vi "Seq Dialog ParemeterSet2.0.vi"(8 "Segment Data":T1) -> (0 "Step Hisitory":string[](array[string]), 2 "Segment Data 2":T1)   [LabVIEW 2018]
uses:
  type defs/Sequence Info.ctl
  type defs/17x Audit Motion Data Seq Control.ctl
  type defs/17x AP Data Type.ctl
panel:
  out "String":string="Pre Run Station - Glass - Vent Open"
  out "error out":errorcluster
  out "value":T2={"Power Supply Voltage"=0.0, "Min Avg Current"=0.0, "Max Avg Current"=0.0, "Min Run Time"=0.0, "Max Run Time"=0.0, "Min Speed"=0.0, "Max Speed"=0.0, "AP Data % of Threshold"=10.0, "Travel Distance"=0.0, "AP Data Type"=enum."91/61", "Check Current"=FALSE, "Check Run Time"=FALSE, "Check Speed"=FALSE, "Express Motion?"=FALSE, "Check Sound Test"=FALSE, "Check Position?"=FALSE, "Collect AP Data"=FALSE, "Inital Position"=0, "End Position"=0, "Goto Posiition"=0, "Max max Current"=0.0, "Min max Current"=0.0, "Check max Current"=FALSE, "Check Sound"=FALSE, "Min Sound (dB)"=0.0, "Max Sound (dB)"=0.0, "SW Mode"=enum."Hard Switch", "LIN Msg"={"ID"=0, "Msg"=[], "LDF"="EX1H"}} {"LIN Msg"."Msg" format="%02x"; "LIN Msg"."ID" format="%02x"}
  in  "Description":string
  in  "Save":bool
  in  "Cancel":bool
  in  "Goto Position":u16=133 max=6750
  in  "FullClose Position":u16=133 min=80 max=6750
  in  "FullOpen Position":u16=133 min=80 max=6750
  in  "Check max Current":bool
  in  "Max max Current (amps)":dbl=10.0
  in  "Min max Current (amps)":dbl=10.0
  in  "Max Speed (mm/sec)":dbl=10.0
  in  "Min Speed (mm/sec)":dbl=10.0
  in  "Check Speed":bool
  in  "Travel Distance (mm)":dbl=133.0
  in  "Check Current":bool
  in  "Check Run Time":bool
  in  "Max Run Time (secs)":dbl=10.0
  in  "Min Run Time (secs)":dbl=10.0
  in  "Max Avg Current (amps)":dbl=10.0
  in  "Min Avg Current (amps)":dbl=10.0
  in  "Power Supply Voltage (V)":dbl=13.0
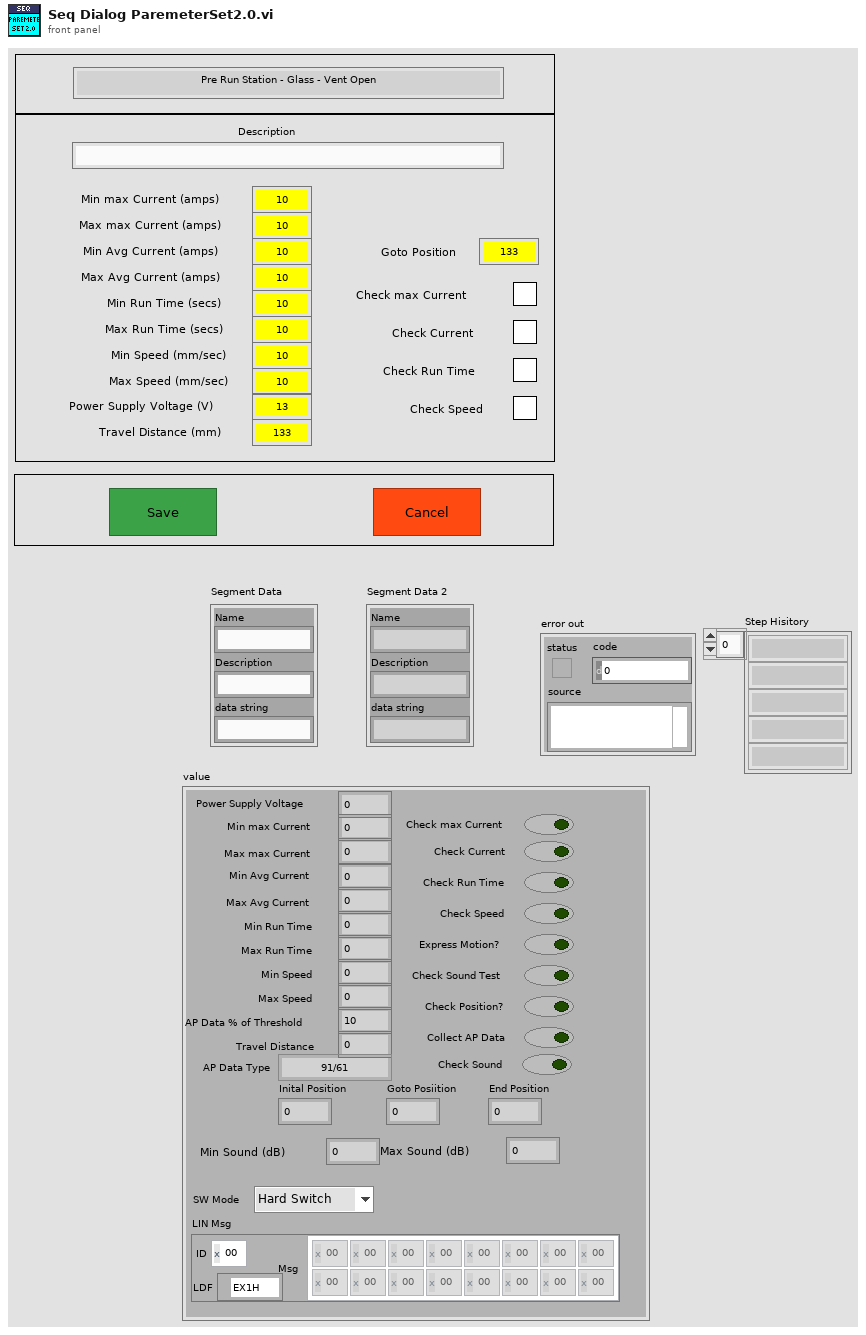
[diagram p1: front panel]
types:
  T1 = typedef "Sequence Info.ctl" = cluster{"Name":string, "Description":string, "data string":string}
  T2 = typedef "17x Audit Motion Data Seq Control.ctl" = cluster{"Power Supply Voltage":dbl, "Min Avg Current":dbl, "Max Avg Current":dbl, "Min Run Time":dbl, "Max Run Time":dbl, "Min Speed":dbl, "Max Speed":dbl, "AP Data % of Threshold":dbl, "Travel Distance":dbl, "AP Data Type":T3, "Check Current":bool, "Check Run Time":bool, "Check Speed":bool, "Express Motion?":bool, "Check Sound Test":bool, "Check Position?":bool, "Collect AP Data":bool, "Inital Position":u16, "End Position":u16, "Goto Posiition":u16, "Max max Current":dbl, "Min max Current":dbl, "Check max Current":bool, "Check Sound":bool, "Min Sound (dB)":dbl, "Max Sound (dB)":dbl, "SW Mode":enum16{"Hard Switch", "Uncond Frame"}, "LIN Msg":cluster{"ID":u8, "Msg":u8[][], "LDF":refnum<k21>}}
  T3 = typedef "17x AP Data Type.ctl" = enum16{"91/61", "92/62", "93/63", "67", "68", "6F", "71", "91 Msg", "92 Msg", "93 Msg", "94 Msg", "HiRain 91", "HiRain 92 Speed", "HiRain 92 HS", "HiRain 92", "HiRain 93", "SnT"}
  T4 = cluster{"Hall Positions":i32[], "Hall path":path, "Motion Data Cluster":T2, "Segment Data":T1, "Old Data":string, "New Data":string}
  T5 = typedef "config paths for seq def.ctl" = cluster{"Part Type":string, "base path":path}
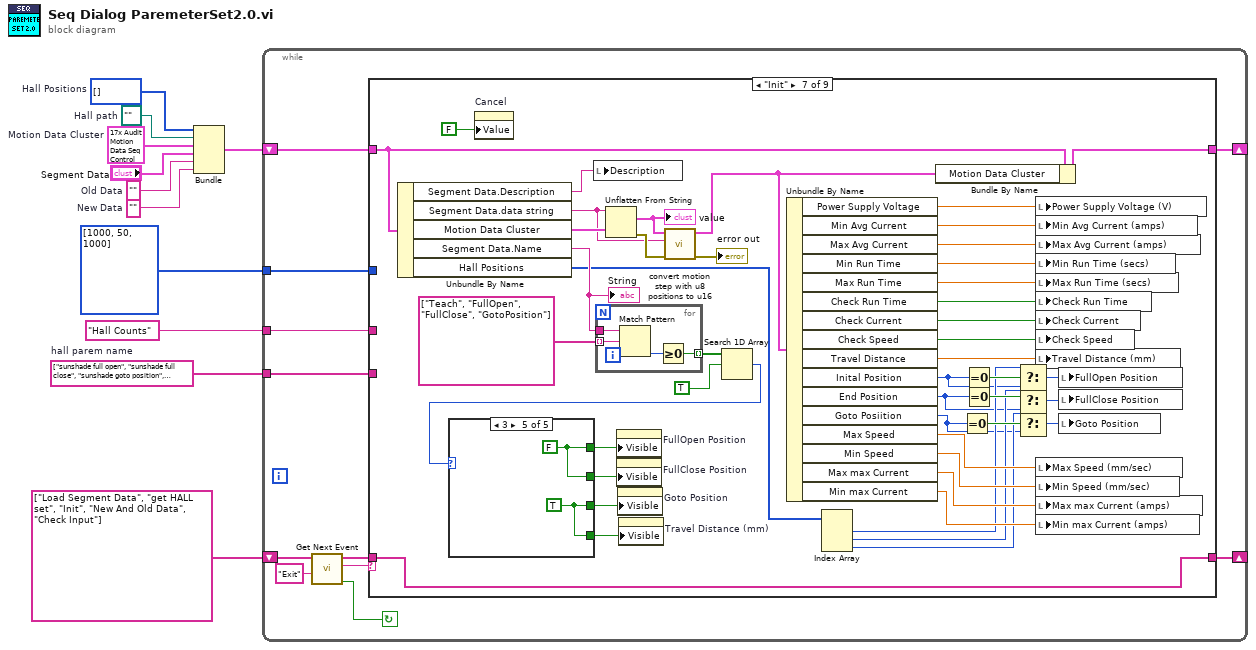
[diagram p0: block diagram]
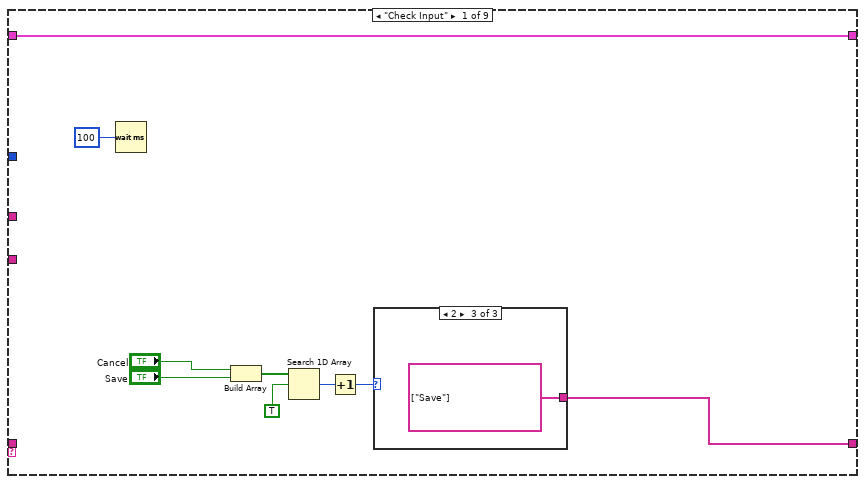
[diagram p2: hidden frame]
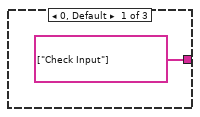
[diagram p3: hidden frame]
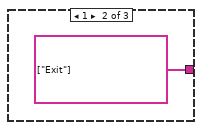
[diagram p4: hidden frame]
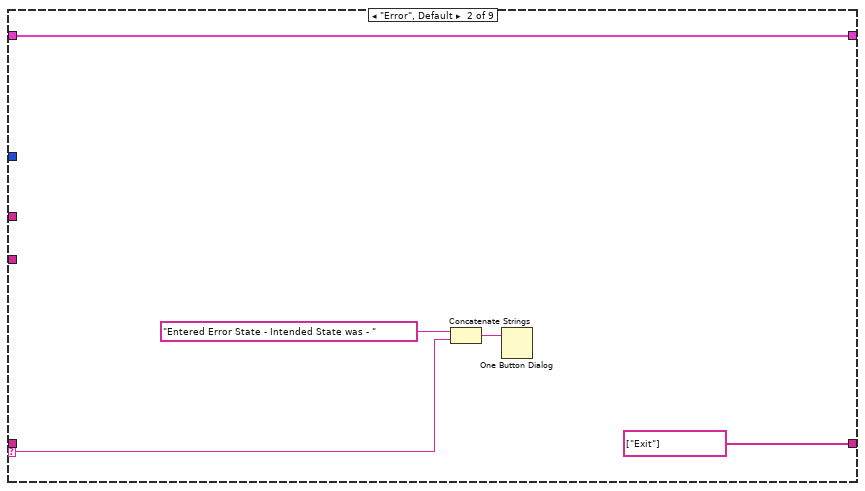
[diagram p5: hidden frame]
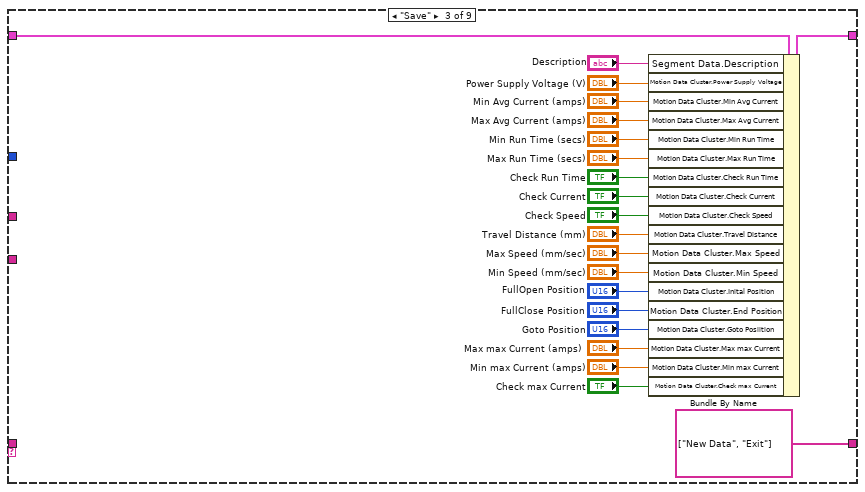
[diagram p6: hidden frame]
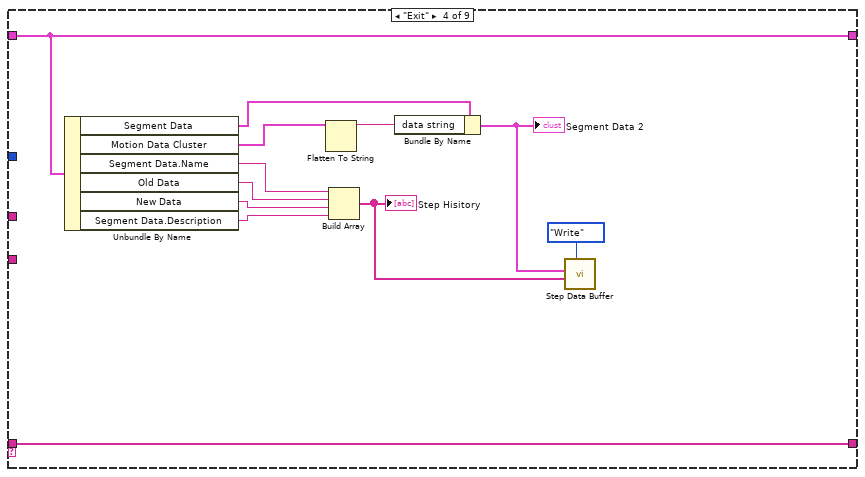
[diagram p7: hidden frame]
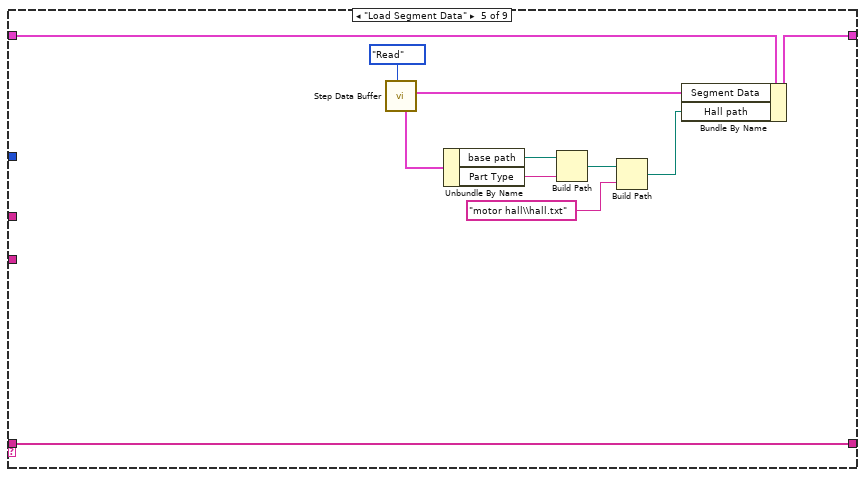
[diagram p8: hidden frame]
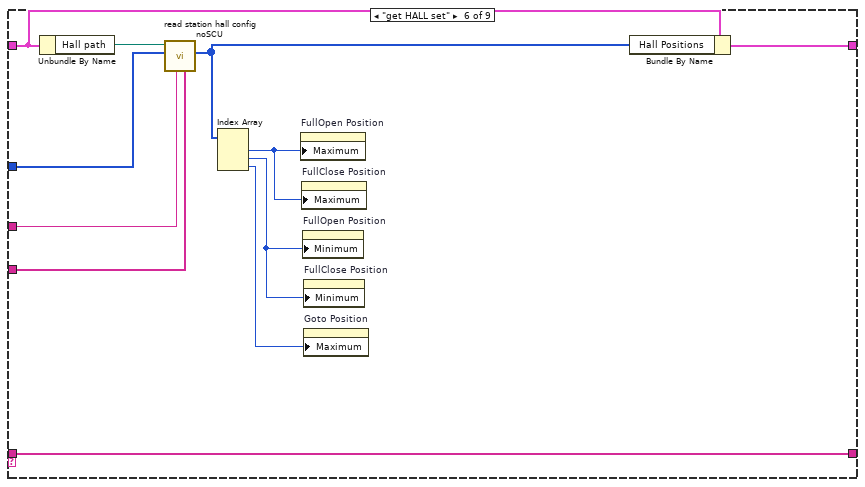
[diagram p9: hidden frame]
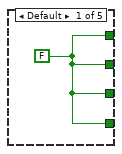
[diagram p10: hidden frame]
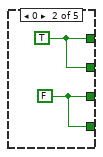
[diagram p11: hidden frame]
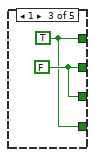
[diagram p12: hidden frame]
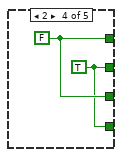
[diagram p13: hidden frame]
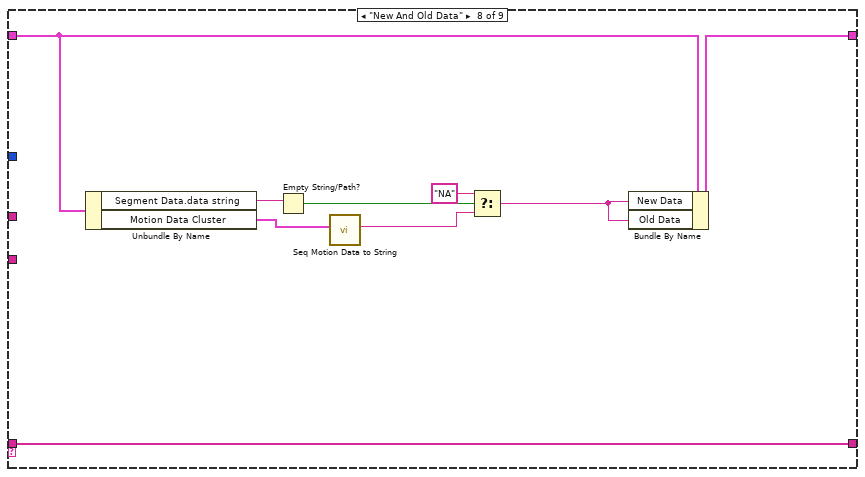
[diagram p14: hidden frame]
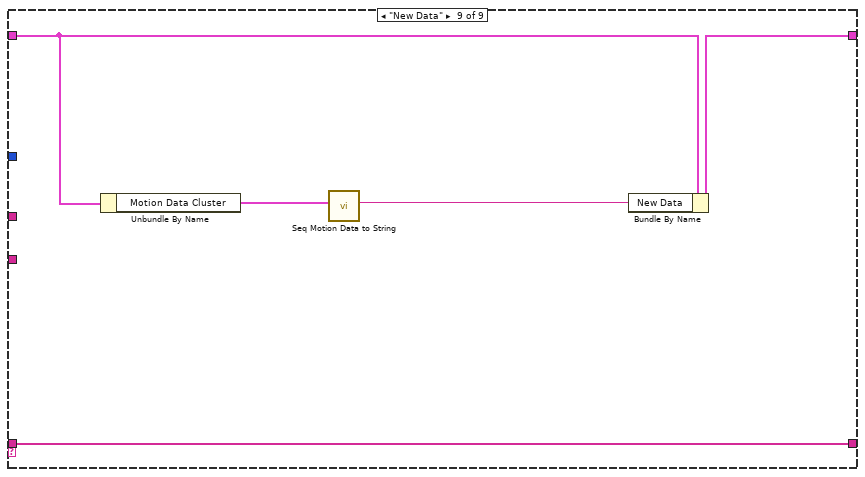
[diagram p15: hidden frame]
diagram:
  w5 = path ""  # Hall path
  w1 = string[] ["sunshade full open", "sunshade full close", "sunshade goto position", "sunshade open drift offset", "sunshade close drift offset", "sunshade goto position drift offset"]  # hall parem name
  w4 = i32[] []  # Hall Positions
  w10 = T2 {"Power Supply Voltage"=0.0, "Min Avg Current"=0.0, "Max Avg Current"=0.0, "Min Run Time"=0.0, "Max Run Time"=0.0, "Min Speed"=0.0, "Max Speed"=0.0, "AP Data % of Threshold"=0.0, "Travel Distance"=0.0, "AP Data Type"=enum."91/61", "Check Current"=FALSE, "Check Run Time"=FALSE, "Check Speed"=FALSE, "Express Motion?"=FALSE, "Check Sound Test"=FALSE, "Check Position?"=FALSE, "Collect AP Data"=FALSE, "Inital Position"=0, "End Position"=0, "Goto Posiition"=0, "Max max Current"=0.0, "Min max Current"=0.0, "Check max Current"=FALSE, "Check Sound"=FALSE, "Min Sound (dB)"=0.0, "Max Sound (dB)"=0.0, "SW Mode"=enum."Hard Switch", "LIN Msg"={"ID"=0, "Msg"=[], "LDF"="EX1H"}}  # Motion Data Cluster
  w7 = ""  # New Data
  w8 = ""  # Old Data
  n1 = Bundle("Hall Positions"=w4, "Hall path"=w5, "Motion Data Cluster"=w10, "Segment Data"="Segment Data", "Old Data"=w8, "New Data"=w7) -> (w11:T4)  [unwired: 1 in]
  n2 = while {
    shift-right: [w20] -> _
    shift-left: string[] ["Load Segment Data", "get HALL set", "Init", "New And Old Data", "Check Input"] ("Event queue out") -> [w19]
    shift-right: [w15] -> _
    shift-left: w11 -> [w16]
    tunnel: i32[] [1000, 50, 1000] ("Hall Positions") -> [w14]
    tunnel: "Hall Counts" ("section") -> [w13]
    tunnel: w1 -> [w12]
    stop <- w18 continue-if-true
    n3 = call "Get Next Event.vi"("Exit Event"="Exit", "event queue in"=w19) -> ("Condition (Exit:F)"=w18:bool, "next event"=w22:string, "event queue out"=w21:string[])  [unwired: 3 in]
    n4 = case shown="\"Init\"" w22 {
      selector: w22 -> [_ w36 _ _ _ _ _ _ _]
      tunnel: w21 -> [_ _ _ w72 w82 w84 w96 w162 w167]
      tunnel: [w25 string[] ["Exit"] ("event queue out") string[] ["New Data", "Exit"] ("Event queue out") w72 w82 w84 w96 w162 w167] -> w20
      tunnel: w16 -> [w31 w35 w60 w68 w81 w92 w138 w157 w166]
      tunnel: [w31 w35 w59 w68 w80 w90 w137 w156 w165] -> w15
      tunnel: w14 -> [_ _ _ _ _ w93 _ _ _]
      tunnel: w13 -> [_ _ _ _ _ w86 _ _ _]
      tunnel: w12 -> [_ _ _ _ _ w85 _ _ _]
      frame "Check Input" {
        n5 = Wait (ms)(milliseconds to wait=u32 100) -> ()  [unwired: 1 out]
        n6 = Build Array("Cancel", "Save") -> (w27:bool[])
        n7 = Search 1D Array(1D array=w27, element=TRUE) -> (index of element=w28:i32)  [unwired: 1 in]
        n8 = Increment(x=w28) -> (x+1=w29:i32)
        n9 = case shown="2" w29 {
          tunnel: [string[] ["Check Input"] ("Events to Insert") string[] ["Exit"] ("Events to Insert") string[] ["Save"] ("Events to Insert")] -> w25
          frame 0, Default {
          }
          frame 1 {
          }
          frame 2 {
          }
        }
      }
      frame "Error", Default {
        n10 = Concatenate Strings("Entered Error State - Intended State was - " ("string"), w36) -> (w38:string)
        n11 = One Button Dialog(message=w38) -> ()  [unwired: 1 in, 1 out]
      }
      frame "Save" {
        n12 = Bundle By Name(cluster=w60, "Segment Data.Description"="Description", "Motion Data Cluster.Power Supply Voltage"="Power Supply Voltage (V)", "Motion Data Cluster.Min Avg Current"="Min Avg Current (amps)", "Motion Data Cluster.Max Avg Current"="Max Avg Current (amps)", "Motion Data Cluster.Min Run Time"="Min Run Time (secs)", "Motion Data Cluster.Max Run Time"="Max Run Time (secs)", "Motion Data Cluster.Check Run Time"="Check Run Time", "Motion Data Cluster.Check Current"="Check Current", "Motion Data Cluster.Check Speed"="Check Speed", "Motion Data Cluster.Travel Distance"="Travel Distance (mm)", "Motion Data Cluster.Max Speed"="Max Speed (mm/sec)", "Motion Data Cluster.Min Speed"="Min Speed (mm/sec)", "Motion Data Cluster.Inital Position"="FullOpen Position", "Motion Data Cluster.End Position"="FullClose Position", "Motion Data Cluster.Goto Posiition"="Goto Position", "Motion Data Cluster.Max max Current"="Max max Current (amps)", "Motion Data Cluster.Min max Current"="Min max Current (amps)", "Motion Data Cluster.Check max Current"="Check max Current") -> (w59:T4)
      }
      frame "Exit" {
        n13 = Unbundle By Name(w68) -> ("Segment Data"=w66:T1, "Motion Data Cluster"=w67:T2, "Segment Data.Name"=w70:string, "Old Data"=w69:string, "New Data"=w71:string, "Segment Data.Description"=w61:string)
        n14 = Flatten To String(anything=w67) -> (data string=w65:string)  [unwired: 3 in, 2 out]
        n15 = Build Array(w70, w69, w71, w61) -> (w62:string[])
        "Step Hisitory" <- w62
        n16 = Bundle By Name(cluster=w66, "data string"=w65) -> (w63:T1)
        "Segment Data 2" <- w63
        n17 = call "Step Data Buffer.vi"("Mode"=enum16{"Init", "Read", "Write"}."Write", "Step Hisitory In"=w62, "Segment Data In"=w63) -> ()  [unwired: 4 in, 5 out]
      }
      frame "Load Segment Data" {
        n18 = call "Step Data Buffer.vi"("Mode"=enum16{"Init", "Read", "Write"}."Read") -> ("Segment Data Out"=w79:T1, "config paths"=w74:T5)  [unwired: 6 in, 3 out]
        n19 = Unbundle By Name(w74) -> ("base path"=w78:path, "Part Type"=w77:string)
        n20 = Build Path(base path=w78, name or relative path=w77) -> (appended path=w76:path)
        n21 = Build Path(base path=w76, name or relative path="motor hall\\hall.txt" ("名称或相对路径")) -> (appended path=w73:path)
        n22 = Bundle By Name(cluster=w81, "Segment Data"=w79, "Hall path"=w73) -> (w80:T4)
      }
      frame "get HALL set" {
        n23 = Unbundle By Name(w92) -> ("Hall path"=w94:path)
        n24 = call "read station hall config noSCU.vi"("name"=w85, "section"=w86, "default value"=w93, "configuration file path in"=w94) -> ("Hall Positions"=w91:i32[])  [unwired: 4 in, 3 out]
        n25 = Index Array(array=w91) -> (element #1=w89:i32, element #2=w88:i32, element #3=w87:i32)  [unwired: 3 in]
        n26 = property on="FullOpen Position" class="DigNum (严格)"("Maximum"=w89) -> ()  [unwired: 2 in, 2 out]
        n27 = property on="FullClose Position" class="DigNum (严格)"("Maximum"=w89) -> ()  [unwired: 2 in, 2 out]
        n28 = property on="FullOpen Position" class="DigNum (严格)"("Minimum"=w88) -> ()  [unwired: 2 in, 2 out]
        n29 = property on="FullClose Position" class="DigNum (严格)"("Minimum"=w88) -> ()  [unwired: 2 in, 2 out]
        n30 = property on="Goto Position" class="DigNum (严格)"("Maximum"=w87) -> ()  [unwired: 2 in, 2 out]
        n31 = Bundle By Name(cluster=w92, "Hall Positions"=w91) -> (w90:T4)
      }
      frame "Init" {
        n32 = Unbundle By Name(w138) -> ("Segment Data.Description"=w139:string, "Segment Data.data string"=w122:string, "Motion Data Cluster"=w140:T2, "Segment Data.Name"=w117:string, "Hall Positions"=w109:i32[])
        "String" <- w117
        n33 = property on="Cancel" class="Bool (严格)"("Value"=FALSE ("Cancel")) -> ()  [unwired: 2 in, 2 out]
        n34 = local write "Description"(w139) -> ()
        n35 = for {
          tunnel: w117 -> [w153]
          tunnel: string[] ["Teach", "FullOpen", "FullClose", "GotoPosition"] -> [w152] mode=indexing
          tunnel: [w150] -> w115 mode=indexing
          n36 = Match Pattern(string=w153, regular expression=w152) -> (offset past match=w151:i32)  [unwired: 1 in, 3 out]
          n37 = Greater Or Equal To 0?(x=w151) -> (x >= 0?=w150:bool)
        }
        n38 = Unflatten From String(type=w140, binary string=w122) -> (value=w121:T2, error out=w124:errorcluster)  [unwired: 3 in, 1 out]
        "value" <- w121
        n39 = call "convert motion step with u8 positions to u16.vi"("error in"=w124, "data string"=w122, "Motion Data Cluster in"=w121) -> ("error out"=→"error out":errorcluster, "Motion Data Cluster out"=w120:T2)  [unwired: 7 in]
        n40 = Search 1D Array(1D array=w115, element=TRUE ("元素")) -> (index of element=w113:i32)  [unwired: 1 in]
        n41 = case shown="3" w113 {
          tunnel: [w141 w143 w144 w147 w149] -> w112
          tunnel: [w141 w143 w145 w146 w149] -> w111
          tunnel: [w141 w142 w145 w147 w148] -> w110
          tunnel: [w141 w142 w144 w146 w148] -> w95
          frame Default {
            w141 = FALSE
          }
          frame 0 {
            w142 = FALSE
            w143 = TRUE
          }
          frame 1 {
            w145 = FALSE
            w144 = TRUE
          }
          frame 2 {
            w147 = FALSE
            w146 = TRUE
          }
          frame 3 {
            w148 = TRUE
            w149 = FALSE
          }
        }
        n42 = property on="FullOpen Position" class="DigNum (严格)"("Visible"=w112) -> ()  [unwired: 2 in, 2 out]
        n43 = property on="FullClose Position" class="DigNum (严格)"("Visible"=w111) -> ()  [unwired: 2 in, 2 out]
        n44 = property on="Goto Position" class="DigNum (严格)"("Visible"=w110) -> ()  [unwired: 2 in, 2 out]
        n45 = property on="Travel Distance (mm)" class="DigNum (严格)"("Visible"=w95) -> ()  [unwired: 2 in, 2 out]
        n46 = Unbundle By Name(w120) -> ("Power Supply Voltage"=w136:dbl, "Min Avg Current"=w135:dbl, "Max Avg Current"=w134:dbl, "Min Run Time"=w133:dbl, "Max Run Time"=w132:dbl, "Check Run Time"=w131:bool, "Check Current"=w130:bool, "Check Speed"=w129:bool, "Travel Distance"=w128:dbl, "Inital Position"=w97:u16, "End Position"=w98:u16, "Goto Posiition"=w99:u16, "Max Speed"=w127:dbl, "Min Speed"=w126:dbl, "Max max Current"=w119:dbl, "Min max Current"=w118:dbl)
        n47 = Index Array(array=w109) -> (element #1=w105:i32, element #2=w103:i32, element #3=w102:i32)  [unwired: 3 in]
        n48 = Bundle By Name(cluster=w138, "Motion Data Cluster"=w120) -> (w137:T4)
        n49 = Equal To 0?(x=w99) -> (x = 0?=w106:bool)
        n50 = Equal To 0?(x=w97) -> (x = 0?=w108:bool)
        n51 = Equal To 0?(x=w98) -> (x = 0?=w107:bool)
        n52 = Select(t=w105, s=w108, f=w97) -> (s? t:f=w104:i32)
        n53 = Select(t=w103, s=w107, f=w98) -> (s? t:f=w101:i32)
        n54 = Select(t=w102, s=w106, f=w99) -> (s? t:f=w100:i32)
        n55 = local write "Power Supply Voltage (V)"(w136) -> ()
        n56 = local write "Min Avg Current (amps)"(w135) -> ()
        n57 = local write "Max Avg Current (amps)"(w134) -> ()
        n58 = local write "Min Run Time (secs)"(w133) -> ()
        n59 = local write "Max Run Time (secs)"(w132) -> ()
        n60 = local write "Check Run Time"(w131) -> ()
        n61 = local write "Check Current"(w130) -> ()
        n62 = local write "Check Speed"(w129) -> ()
        n63 = local write "Travel Distance (mm)"(w128) -> ()
        n64 = local write "Max Speed (mm/sec)"(w127) -> ()
        n65 = local write "Min Speed (mm/sec)"(w126) -> ()
        n66 = local write "Max max Current (amps)"(w119) -> ()
        n67 = local write "Min max Current (amps)"(w118) -> ()
        n68 = local write "FullOpen Position"(w104) -> ()
        n69 = local write "FullClose Position"(w101) -> ()
        n70 = local write "Goto Position"(w100) -> ()
      }
      frame "New And Old Data" {
        n71 = Unbundle By Name(w157) -> ("Segment Data.data string"=w161:string, "Motion Data Cluster"=w155:T2)
        n72 = Empty String/Path?(string/path=w161) -> (empty?=w160:bool)
        n73 = call "Seq Motion Data to String.vi"("Motion Data Cluster"=w155) -> ("Data String"=w154:string)  [unwired: 10 in]
        n74 = Select(t="NA", s=w160, f=w154) -> (s? t:f=w158:string)
        n75 = Bundle By Name(cluster=w157, "New Data"=w158, "Old Data"=w158) -> (w156:T4)
      }
      frame "New Data" {
        n76 = Unbundle By Name(w166) -> ("Motion Data Cluster"=w164:T2)
        n77 = call "Seq Motion Data to String.vi"("Motion Data Cluster"=w164) -> ("Data String"=w163:string)  [unwired: 10 in]
        n78 = Bundle By Name(cluster=w166, "New Data"=w163) -> (w165:T4)
      }
    }
  }
